vi "Timestamp_Calculate t0 from tf and size.vi"(7 "Dt":dbl, 10 "Size":i32, 11 "Tf":timestamp) -> (3 "T0 Out":timestamp)   [LabVIEW 2020]
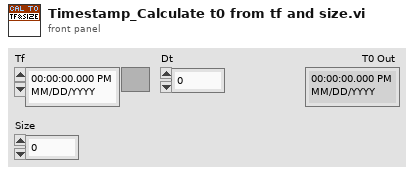
[diagram p1: front panel]
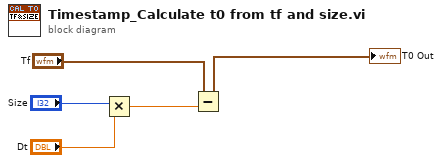
[diagram p0: block diagram]
diagram:
  n1 = Multiply(x="Size", y="Dt") -> (x*y=w2:dbl)
  n2 = Subtract(x="Tf", y=w2) -> (x-y=→"T0 Out":timestamp)
